vi "Parse Identifier.vi"(11 "string":string) -> (1 "found?":bool, 2 "identifier":string, 3 "remaining string":string)   [LabVIEW 2018, in "Logging.lvlib" / "Format String.lvclass"]
uses:
  Format String.lvclass
panel:
  # "Connector Pane"
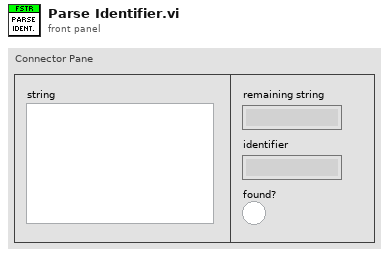
[diagram p1: front panel]
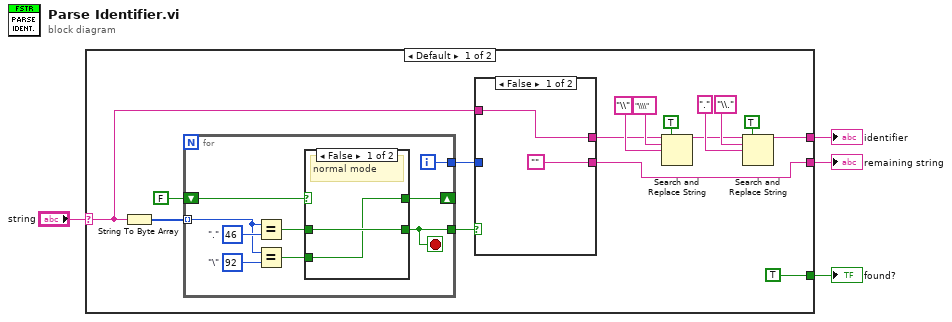
[diagram p0: block diagram]
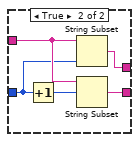
[diagram p2: hidden frame]
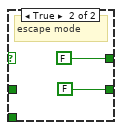
[diagram p3: hidden frame]
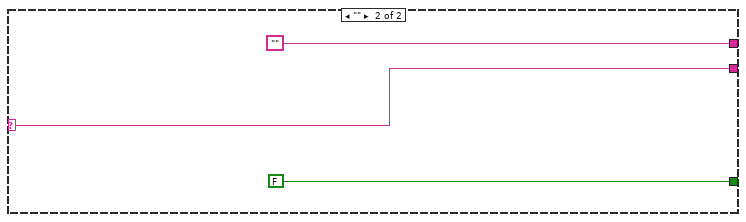
[diagram p4: hidden frame]
diagram:
  n1 = case shown="Default" "string" {
    selector: "string" -> [w17 w43]
    tunnel: [w5 w43] -> w3
    tunnel: [w6 ""] -> w2
    tunnel: [TRUE ("found?") FALSE ("found?")] -> w1
    frame Default {
      n2 = String To Byte Array(string=w17) -> (unsigned byte array=w20:u8[])
      n3 = for {
        tunnel: w20 -> [w33] mode=indexing
        tunnel: [w36] -> w19
        shift-right: [w28] -> _
        shift-left: FALSE -> [w35]
        tunnel: [w29] -> w15
        i -> [w36]
        stop <- w29 stop-if-true
        w32 = u8 92  # "\"
        w34 = u8 46  # "."
        n4 = Equal?(x=w33, y=w34) -> (x = y?=w31:bool)
        n5 = Equal?(x=w33, y=w32) -> (x = y?=w30:bool)
        n6 = case shown="False" w35 {
          tunnel: w31 -> [w38 _]
          tunnel: w30 -> [w37 _]
          tunnel: [w38 FALSE] -> w29
          tunnel: [w37 FALSE] -> w28
          frame False {
            # "normal mode"
          }
          frame True {
            # "escape mode"
          }
        }
      }
      n7 = case shown="False" w15 {
        tunnel: w19 -> [_ w23]
        tunnel: ["" w27] -> w5
        tunnel: w17 -> [w22 w26]
        tunnel: [w22 w24] -> w7
        frame False {
        }
        frame True {
          n8 = Increment(x=w23) -> (x+1=w25:i32)
          n9 = String Subset(string=w26, length (rest)=w23) -> (substring=w24:string)  [unwired: 1 in]
          n10 = String Subset(string=w26, offset (0)=w25) -> (substring=w27:string)  [unwired: 1 in]
        }
      }
      n11 = Search and Replace String(replace all?=TRUE ("replace all? (F)"), input string=w7, search string="\\\\", replace string="\\" ("replace string (\"\")")) -> (result string=w8:string)  [unwired: 4 in, 3 out]
      n12 = Search and Replace String(replace all?=TRUE ("replace all? (F)"), input string=w8, search string="\\.", replace string="." ("replace string (\"\")")) -> (result string=w6:string)  [unwired: 4 in, 3 out]
    }
    frame "" {
    }
  }
  "remaining string" <- w3
  "identifier" <- w2
  "found?" <- w1
